vi "Draw Border.vi"(9 "State":T1) -> (3 "Picture":picture)   [LabVIEW 2020, in "Parallel Diagram Block.xnode"]
uses:
  Parallel Diagram Block.xnode
  State.ctl
  Parallel Block/Type Descriptor.ctl
  Parallel Block/Direction.ctl
  Parallel Block/Value Type.ctl
  Parallel Block/Terminal Mode.ctl
  Parallel Block/Terminal Type.ctl
  <vilib>/picture/picture.llb/imagedata.ctl
  <vilib>/XNodeSupport/XNodeInt.ctl
  <vilib>/XNodeSupport/NI_XNodeSupport.lvlib
  Parallel Block/Parallel Block.lvlib
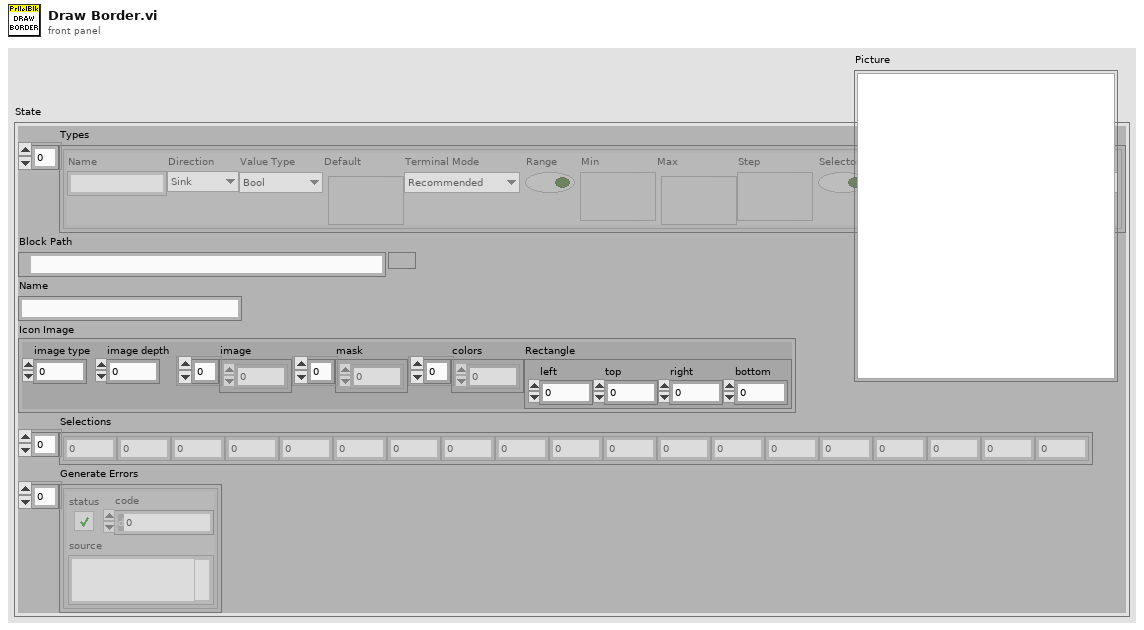
[diagram p1: front panel]
types:
  T1 = typedef "Parallel Diagram Block.xnode/State.ctl" = cluster{"Types":T2[], "Block Path":path, "Name":string, "Icon Image":T7, "Selections":i32[], "Generate Errors":errorcluster[]}
  T2 = typedef "Parallel Block.lvlib/Type Descriptor.ctl" = cluster{"Name":string, "Direction":T3, "Value Type":T4, "Default":variant, "Terminal Mode":T5, "Range":bool, "Min":variant, "Max":variant, "Step":variant, "Selector":bool, "Options":string[], "Terminal Type":T6}
  T3 = typedef "Parallel Block.lvlib/Direction.ctl" = enum16{"Sink", "Source"}
  T4 = typedef "Parallel Block.lvlib/Value Type.ctl" = enum16{"Unknown", "Bool", "U8", "U16", "U32", "U64", "I8", "I16", "I32", "I64", "SGL", "DBL", "CSG", "CDB", "CDBWfm", "String", "DBLWfm"}
  T5 = typedef "Parallel Block.lvlib/Terminal Mode.ctl" = enum16{"Recommended", "Required", "None"}
  T6 = typedef "Parallel Block.lvlib/Terminal Type.ctl" = enum16{"Unwired", "Connection", "Value", "Control Ref"}
  T7 = typedef "imagedata.ctl" = cluster{"image type":i32, "image depth":i32, "image":u8[], "mask":u8[], "colors":u32[], "Rectangle":cluster{"left":i16, "top":i16, "right":i16, "bottom":i16}}
  T8 = typedef "NI_XNodeSupport.lvlib/XNodeBounds.ctl" = cluster{"Width":T9, "Height":T9}
  T9 = typedef "NI_XNodeSupport.lvlib/XNodeInt.ctl" = i32
  T10 = cluster{"left":i16, "top":i16, "right":i16, "bottom":i16}
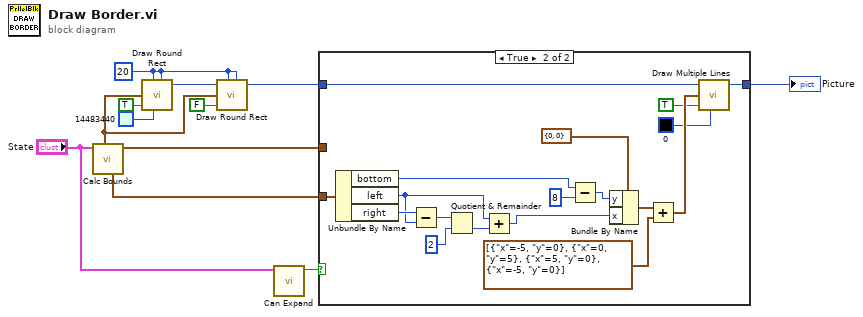
[diagram p0: block diagram]
diagram:
  w8 = i16 20 ("oval width")
  n1 = call "Calc Bounds.vi"("State"="State") -> ("Bounds"=w3:T8, "Bounds Without Terminals"=w4:T10, "Full Bounds"=w1:T10)  [unwired: 6 in, 2 out]
  n2 = call <vilib>:"Draw Round Rect.vi"("oval width"=w8, "rect"=w1, "fill?(F)"=TRUE, "color(black)"=u32 14483440, "oval height"=w8) -> ("new picture"=w10:picture)  [unwired: 4 in]
  n3 = call <vilib>:"Draw Round Rect.vi"("picture"=w10, "oval width"=w8, "rect"=w1, "fill?(F)"=FALSE, "oval height"=w8) -> ("new picture"=w7:picture)  [unwired: 4 in]
  n4 = call "Can Expand.vi"("State"="State") -> ("Can Expand?"=w2:bool)  [unwired: 10 in]
  n5 = case shown="True" w2 {
    tunnel: w7 -> [w13 w25]
    tunnel: [w13 w24] -> w6
    tunnel: w4 -> [_ w16]
    tunnel: w3 -> [_ _]
    frame False {
    }
    frame True {
      n6 = Unbundle By Name(w16) -> ("bottom"=w15:i16, "left"=w17:i16, "right"=w20:i16)
      n7 = Subtract(x=w20, y=w17) -> (x-y=w19:i16)
      n8 = Quotient & Remainder(x=w19, y=2) -> (floor(x/y)=w18:i32)  [unwired: 1 out]
      n9 = Add(x=w17, y=w18) -> (x+y=w14:i32)
      n10 = Subtract(x=w15, y=T9 8) -> (x-y=w29:T9)
      n11 = Bundle By Name(cluster=cluster{"x":i16, "y":i16} {"x"=0, "y"=0}, "y"=w29, "x"=w14) -> (w28:cluster{"x":i16, "y":i16})
      n12 = Add(x=w28, y=cluster{"x":i16, "y":i16}[] [{"x"=-5, "y"=0}, {"x"=0, "y"=5}, {"x"=5, "y"=0}, {"x"=-5, "y"=0}] ("line endpoints")) -> (x+y=w26:cluster{"x":i16, "y":i16}[])
      n13 = call <vilib>:"Draw Multiple Lines.vi"("picture"=w25, "line endpoints"=w26, "fill?(F)"=TRUE, "color(black)"=u32 0) -> ("new picture"=w24:picture)  [unwired: 5 in]
    }
  }
  "Picture" <- w6
